vi "ArmJoystickControl.vi"(0 "Joystick control":T3) -> (1 "TargetPosition":T1=enum."Forward Cargo Hold", 2 "ArmPlanRequest":T2={"Destination"=enum."Forward Cargo Hold", "Preview"=FALSE, "Start"=enum."Forward Cargo Hold", "Fixed Start"=FALSE}, 3 "NewPath":bool)   [LabVIEW 2018]
uses:
  TypeDefs/JoystickControls.ctl
  TypeDefs/ArmPlanRequest.ctl
  TypeDefs/ArmTargetPosition.ctl
  ArgosLib/Signal Processing/TypeDefs/EdgeDetector_Type.ctl
  Global_Var-RefNum/DriversStationData.vi
  ArgosLib/ArgosLib.lvlib
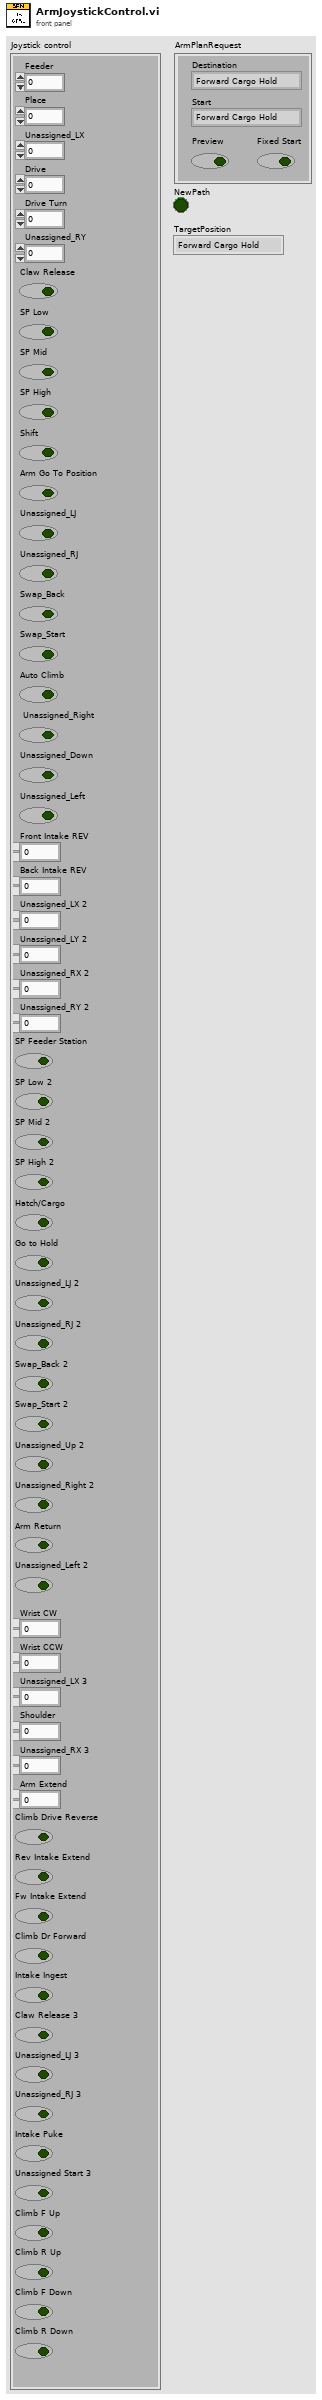
[diagram p1: front panel]
types:
  T1 = typedef "ArmTargetPosition.ctl" = enum16{"Forward Cargo Intake", "Forward Cargo Hold", "Forward Cargo Low", "Forward Cargo Middle", "Forward Cargo High", "Forward Hatch Intake", "Forward Hatch Hold", "Forward Hatch Low", "Forward Hatch Middle", "Forward Hatch High", "Reverse Cargo Intake", "Reverse Cargo Hold", "Reserve Cargo Low", "Reverse Cargo Middle", "Reverse Cargo High", "Reverse Hatch Intake", "Reverse Hatch Hold", "Reverse Hatch Low", "Reverse Hatch Middle", "Reverse Hatch High"}
  T2 = typedef "ArmPlanRequest.ctl" = cluster{"Destination":T1, "Preview":bool, "Start":T1, "Fixed Start":bool}
  T3 = typedef "JoystickControls.ctl" = cluster{"Drive":dbl, "Drive Turn ":dbl, "Unassigned_LX":dbl, "Unassigned_RY":dbl, "Claw Release":bool, "Place":dbl, "Feeder":dbl, "SP Low":bool, "SP Mid":bool, "SP High":bool, "Shift":bool, "Arm Go To Position":bool, "Unassigned_LJ":bool, "Unassigned_RJ":bool, "Swap_Back":bool, "Swap_Start":bool, "Unassigned_LY 2":dbl, "Unassigned_RX 2":dbl, "Unassigned_LX 2":dbl, "Unassigned_RY 2":dbl, "SP Feeder Station":bool, "Back Intake REV":dbl, "Front Intake REV":dbl, "SP Low 2":bool, "SP Mid 2":bool, "SP High 2":bool, "Hatch/Cargo":bool, "Go to Hold":bool, "Unassigned_LJ 2":bool, "Unassigned_RJ 2":bool, "Swap_Back 2":bool, "Swap_Start 2":bool, "Unassigned_Up 2":bool, "Unassigned_Right 2":bool, "Arm Return":bool, "Unassigned_Left 2":bool, "Auto Climb":bool, " Unassigned_Right":bool, "Unassigned_Down":bool, "Unassigned_Left":bool, "Shoulder":dbl, "Unassigned_RX 3":dbl, "Unassigned_LX 3":dbl, "Arm Extend":dbl, "Climb Drive Reverse":bool, "Wrist CCW":dbl, "Wrist CW":dbl, "Rev Intake Extend":bool, "Fw Intake Extend":bool, "Climb Dr Forward":bool, "Intake Ingest ":bool, "Claw Release 3":bool, "Unassigned_LJ 3":bool, "Unassigned_RJ 3":bool, "Intake Puke":bool, "Unassigned Start 3":bool, "Climb F Up":bool, "Climb R Up":bool, "Climb F Down":bool, "Climb R Down":bool}
  T4 = typedef "ArgosLib.lvlib/EdgeDetector_Type.ctl" = enum16{"RisingEdge", "FallingEdge", "Both"}
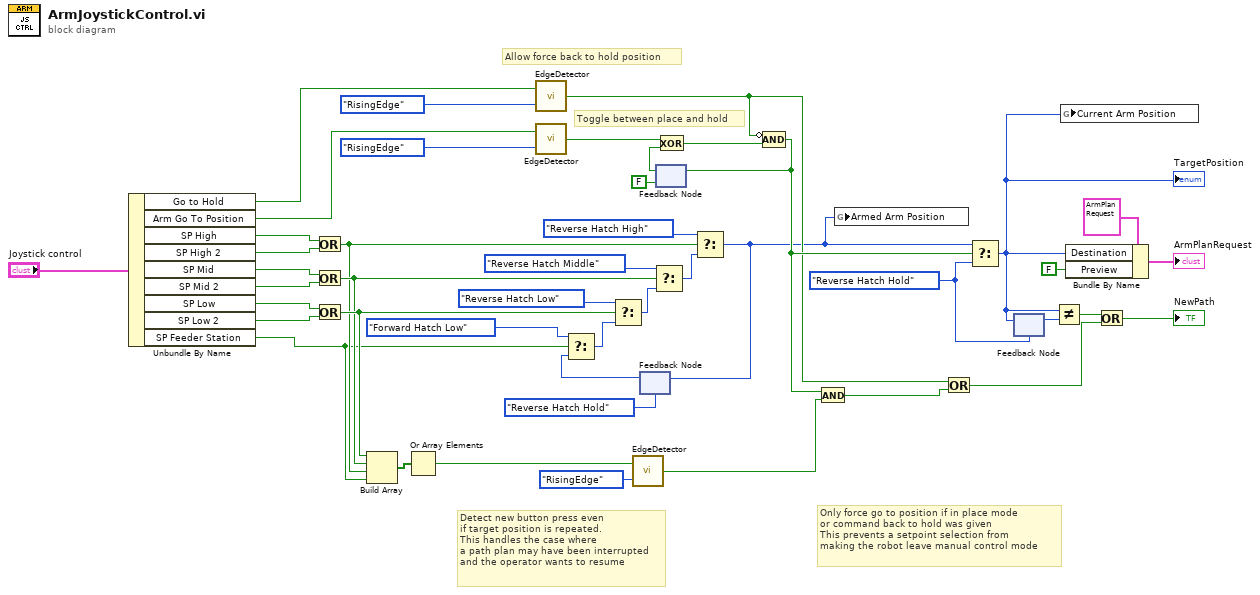
[diagram p0: block diagram]
diagram:
  w28 = ArmTargetPosition."Reverse Hatch Hold" ("f")
  # "Only force go to position if in place mode\nor command back to hold was given\nThis prevents a setpoint selection from\nmaking the robot leave manual control mode"
  # "Allow force back to hold position"
  # "Detect new button press even\nif target position is repeated.\nThis handles the case where\na path plan may have been interrupted\nand the operator wants to resume"
  # "Toggle between place and hold"
  n1 = Unbundle By Name("Joystick control") -> ("Go to Hold"=w17:bool, "Arm Go To Position"=w36:bool, "SP High"=w44:bool, "SP High 2"=w43:bool, "SP Mid"=w42:bool, "SP Mid 2"=w41:bool, "SP Low"=w40:bool, "SP Low 2"=w39:bool, "SP Feeder Station"=w1:bool)
  n2 = Or(x=w44, y=w43) -> (x .or. y?=w23:bool)
  n3 = Or(x=w42, y=w41) -> (x .or. y?=w24:bool)
  n4 = Or(x=w40, y=w39) -> (x .or. y?=w25:bool)
  n5 = Build Array(w25, w24, w23, w1) -> (w22:bool[])
  n6 = Or Array Elements(Boolean array=w22) -> (logical OR=w20:bool)
  n7 = call "EdgeDetector.vi"("DetectorType"=EdgeDetector_Type."RisingEdge", "Input"=w17) -> ("Edge"=w12:bool)
  n8 = call "EdgeDetector.vi"("DetectorType"=EdgeDetector_Type."RisingEdge", "Input"=w36) -> ("Edge"=w32:bool)
  n9 = call "EdgeDetector.vi"("DetectorType"=EdgeDetector_Type."RisingEdge", "Input"=w20) -> ("Edge"=w14:bool)
  n10 = feedback #1(ArmTargetPosition."Reverse Hatch Hold" ("t")) -> (w9:T1)
  n11 = Select(t=ArmTargetPosition."Forward Hatch Low", s=w1, f=w9) -> (s? t:f=w10:T1)
  n12 = Select(t=ArmTargetPosition."Reverse Hatch Low", s=w25, f=w10) -> (s? t:f=w37:T1)
  n13 = Select(t=ArmTargetPosition."Reverse Hatch Middle", s=w24, f=w37) -> (s? t:f=w38:T1)
  n14 = feedback #2(FALSE) -> (w34:bool)
  n15 = Exclusive Or(1:w34, 2:w32) -> (0:w16:bool)
  n16 = Select(t=ArmTargetPosition."Reverse Hatch High", s=w23, f=w38) -> (s? t:f=w3:T1)
  n17 = feedback-in #1(w3) -> ()
  n18 = Compound Arithmetic op=AND(invert w12, w16) -> (w15:bool)
  n19 = feedback-in #2(w15) -> ()
  n20 = And(x=w15, y=w14) -> (x .and. y?=w13:bool)
  n21 = global write "DriversStationData.vi" "Armed Arm Position"(w3) -> ()
  n22 = Or(x=w12, y=w13) -> (x .or. y?=w11:bool)
  n23 = Select(t=w3, s=w15, f=w28) -> (s? t:f=w2:T1)
  "TargetPosition" <- w2
  n24 = feedback-in #3(w2) -> ()
  n25 = feedback #3(w28) -> (w27:T1)
  n26 = Not Equal?(x=w2, y=w27) -> (x != y?=w26:bool)
  n27 = global write "DriversStationData.vi" "Current Arm Position"(w2) -> ()
  n28 = Bundle By Name(cluster=T2 {"Destination"=enum."Forward Cargo Hold", "Preview"=FALSE, "Start"=enum."Forward Cargo Hold", "Fixed Start"=FALSE} ("ArmPlanRequest"), "Destination"=w2, "Preview"=FALSE) -> (→"ArmPlanRequest":T2)
  n29 = Or(x=w26, y=w11) -> (x .or. y?=→"NewPath":bool)
